vi "Connect.vi"(8 "error in (no error)":errorcluster, 11 "VISA TCP in":refnum<class "VISA TCP.lvclass">) -> (0 "error out":errorcluster, 3 "VISA TCP out":refnum<class "VISA TCP.lvclass">)   [LabVIEW 2021, in "Sockets.lvlib" / "VISA TCP.lvclass"]
doc: "Reads data from a socket connection."
uses:
  VISA TCP.lvclass
  VISA TCP.lvclass/VISA TCP.ctl
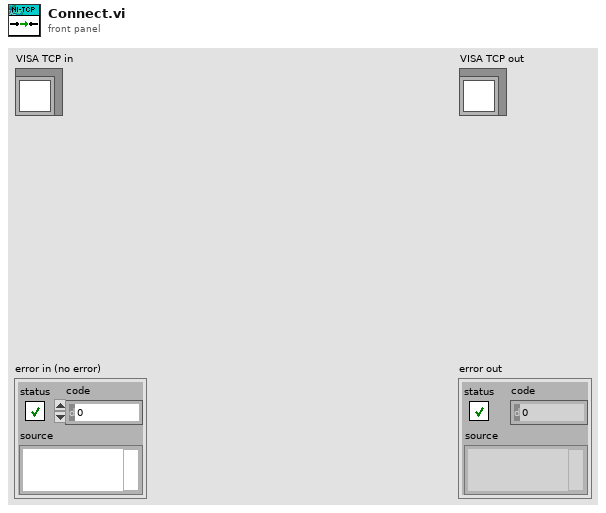
[diagram p1: front panel]
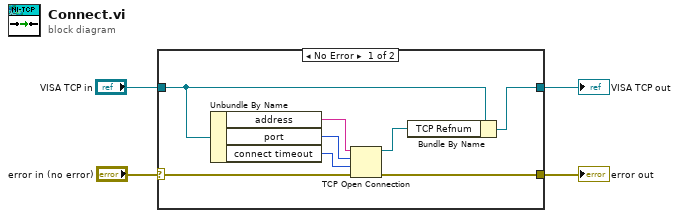
[diagram p0: block diagram]
diagram:
  n1 = case shown="No Error" "error in (no error)" {
    selector: "error in (no error)" -> [w6 w13]
    tunnel: [w10 w13] -> w1
    tunnel: "VISA TCP in" -> [w9 w14]
    tunnel: [w7 w14] -> w3
    frame No Error {
      n2 = Unbundle By Name(w9) -> ("address"=w12:string, "port"=w11:u16, "connect timeout"=w5:i32)
      n3 = TCP Open Connection(address=w12, remote port or service name=w11, timeout ms (60000)=w5, error in (no error)=w6) -> (connection ID=w8:refnum<k5>, error out=w10:errorcluster)  [unwired: 1 in]
      n4 = Bundle By Name(cluster=w9, "TCP Refnum"=w8) -> (w7:refnum<class "VISA TCP.lvclass">)
    }
    frame Error {
    }
  }
  "error out" <- w1
  "VISA TCP out" <- w3
